vi "ClearXYZTheta Go.vi"(8 "error in (no error)":errorcluster, 10 "XYZTheta In":dbl[](array[numeric]), 11 "Gantry In":refnum<k24>) -> (0 "error out":errorcluster, 2 "XYZTheta Out":dbl[](array[numeric]), 3 "Gantry Out":refnum<k24>)   [LabVIEW 2020, in "Motion.lvclass"]
uses:
  Motion.lvclass
  A3200/A3200.lvclass
  Drivers/Aerotech A3200/Aerotech.lvlib
  C:/Program Files (x86)/Aerotech/A3200/LabVIEW/2010/Bin/Aerotech.A3200.dll
  Program Files (x86)/Aerotech/A3200/LabVIEW/2010/Bin/Aerotech.A3200.dll
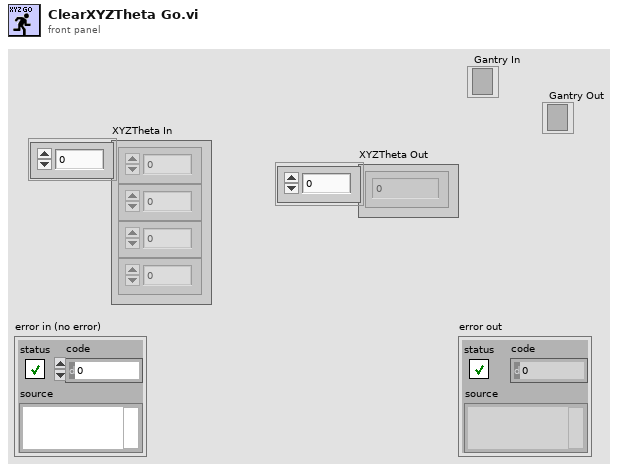
[diagram p1: front panel]
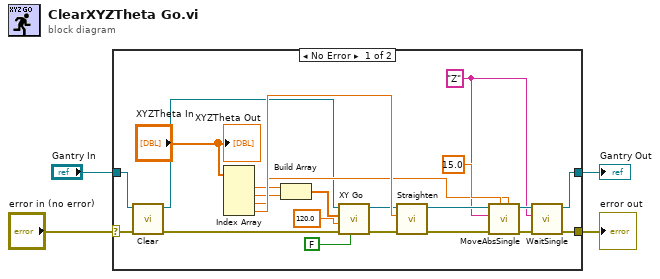
[diagram p0: block diagram]
diagram:
  n1 = case shown="No Error" "error in (no error)" {
    selector: "error in (no error)" -> [w10 w28]
    tunnel: [w6 w28] -> w3
    tunnel: "Gantry In" -> [w12 w27]
    tunnel: [w14 w27] -> w1
    frame No Error {
      w13 = "Z" ("axis name")
      n2 = call "Clear.vi"("error in (no error)"=w10, "Gantry In"=w12) -> ("error out"=w9:errorcluster, "Gantry Out"=w11:refnum<k24>)  [unwired: 8 in]
      n3 = Index Array(array="XYZTheta In") -> (element #1=w22:dbl, element #2=w21:dbl, element #3=w17:dbl, element #4=w24:dbl)  [unwired: 4 in]
      n4 = Build Array(w22, w21) -> (w23:dbl[])
      n5 = call "XY Go.vi"("return immediately"=FALSE, "error in (no error)"=w9, "Speed"=120.0, "XY In"=w23, "Gantry In"=w11) -> ("error out"=w20:errorcluster, "Gantry Out"=w5:refnum<k24>)  [unwired: 4 in, 1 out]
      n6 = call "Straighten.vi"("error in (no error)"=w20, "Angle (rad)"=w24, "Gantry In"=w5) -> ("error out"=w16:errorcluster, "Gantry Out"=w19:refnum<k24>)  [unwired: 7 in]
      n7 = call "MoveAbsSingle.vi"("position"=w17, "speed"=15.0, "error in (no error)"=w16, "axis name"=w13, "controller in"=w19) -> ("error out"=w7:errorcluster, "controller out"=w15:refnum<k24>)  [unwired: 5 in]
      n8 = call "WaitSingle.vi"("error in (no error)"=w7, "axis name"=w13, "controller in"=w15) -> ("error out"=w6:errorcluster, "controller out"=w14:refnum<k24>)  [unwired: 6 in, 1 out]
      "XYZTheta Out" <- "XYZTheta In"
    }
    frame Error {
    }
  }
  "error out" <- w3
  "Gantry Out" <- w1
